vi "BuildAll.vi"   [LabVIEW 2017]
uses:
  <vilib>/AppBuilder/AB_API_Simple/NI_App_Builder_API.lvlib
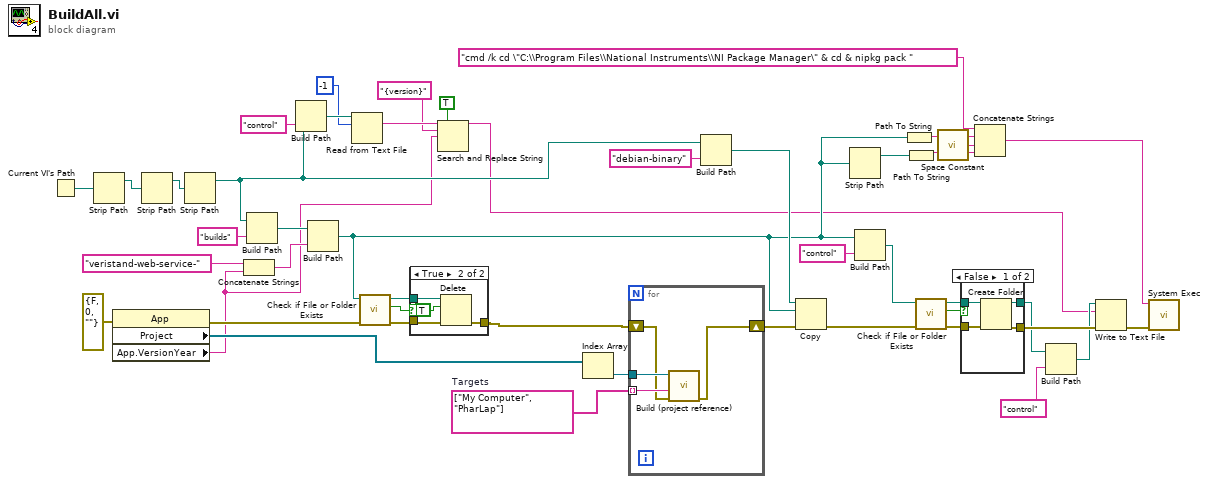
[diagram p0: block diagram]
diagram:
  w44 = string[] ["My Computer", "PharLap"]  # Targets
  n1 = Current VI's Path() -> (path=w42:path)
  n2 = Strip Path(path=w42) -> (stripped path=w41:path)  [unwired: 1 out]
  n3 = property class="App"(error in=errorcluster {"status"=FALSE, "code"=0, "source"=""} ("error in (no error)")) -> (error out=w32:errorcluster, "Project"=w46:refnum<vi>[], "App.VersionYear"=w1:string)  [unwired: 1 in, 1 out]
  n4 = Strip Path(path=w41) -> (stripped path=w27:path)  [unwired: 1 out]
  n5 = Strip Path(path=w27) -> (stripped path=w26:path)  [unwired: 1 out]
  n6 = Concatenate Strings("veristand-web-service-" ("string"), w1) -> (w9:string)
  n7 = Build Path(base path=w26, name or relative path="builds") -> (appended path=w39:path)
  n8 = Build Path(base path=w26, name or relative path="control") -> (appended path=w13:path)
  n9 = Build Path(base path=w39, name or relative path=w9) -> (appended path=w20:path)
  n10 = Read from Text File(file (use dialog)=w13, count=-1) -> (text=w11:string)  [unwired: 2 in, 3 out]
  n11 = call <vilib>:"Check if File or Folder Exists.vi"("error in (no error)"=w32, "path"=w20) -> ("error out"=w31:errorcluster, "file or folder exists?"=w29:bool, "dup path"=w30:path)  [unwired: 7 in]
  n12 = case shown="True" w29 {
    tunnel: w31 -> [w47 w50]
    tunnel: w30 -> [_ w49]
    tunnel: [w47 w48] -> w28
    frame False {
    }
    frame True {
      n13 = Delete(path (use dialog)=w49, entire hierarchy (F)=TRUE, error in=w50) -> (error out=w48:errorcluster)  [unwired: 2 in, 2 out]
    }
  }
  n14 = Search and Replace String(replace all?=TRUE ("replace all? (F)"), input string=w11, search string="{version}", replace string=w1) -> (result string=w2:string)  [unwired: 4 in, 3 out]
  n15 = Index Array(array=w46) -> (element=w45:refnum<vi>)  [unwired: 1 in]
  n16 = for {
    tunnel: w45 -> [w55]
    tunnel: w44 -> [w54] mode=indexing
    shift-right: [w52] -> w35
    shift-left: w28 -> [w53]
    n17 = call <vilib>:"Build (project reference).vi"("error in (no error)"=w53, "Name of target (My Computer)"=w54, "Project reference"=w55) -> ("error out"=w52:errorcluster)  [unwired: 6 in, 2 out]
  }
  n18 = Build Path(base path=w26, name or relative path="debian-binary") -> (appended path=w34:path)
  n19 = Copy(8:w35, 10:w20, 11:w34) -> (0:w23:errorcluster)  [unwired: 2 in, 2 out]
  n20 = Strip Path(path=w20) -> (stripped path=w19:path)  [unwired: 1 out]
  n21 = Build Path(base path=w20, name or relative path="control") -> (appended path=w25:path)
  n22 = Path To String(path=w20) -> (string=w18:string)
  n23 = Path To String(path=w19) -> (string=w15:string)
  n24 = call <vilib>:"Check if File or Folder Exists.vi"("error in (no error)"=w23, "path"=w25) -> ("error out"=w22:errorcluster, "file or folder exists?"=w24:bool, "dup path"=w21:path)  [unwired: 7 in]
  n25 = call <vilib>:"Space Constant.vi"() -> ("String"=w16:string)
  n26 = case shown="False" w24 {
    tunnel: w22 -> [w59 w60]
    tunnel: w21 -> [w58 w61]
    tunnel: [w57 w61] -> w5
    tunnel: [w56 w60] -> w7
    frame False {
      n27 = Create Folder(path (use dialog)=w58, error in=w59) -> (created path=w57:path, error out=w56:errorcluster)  [unwired: 1 in, 1 out]
    }
    frame True {
    }
  }
  n28 = Concatenate Strings("cmd /k cd \"C:\\Program Files\\National Instruments\\NI Package Manager\" & cd & nipkg pack " ("command line"), w18, w16, w15) -> (w14:string)
  n29 = Build Path(base path=w5, name or relative path="control") -> (appended path=w3:path)
  n30 = Write to Text File(file (use dialog)=w3, text=w2, error in=w7) -> (error out=w6:errorcluster)  [unwired: 1 in, 2 out]
  n31 = call <vilib>:"System Exec.vi"("error in (no error)"=w6, "command line"=w14) -> ()  [unwired: 6 in, 4 out]
